vi "Idot Recorder.vi"() -> ()   [LabVIEW 2015]
uses:
  Libraries/NI-DAQ/NI-DAQ digitizer parameters.ctl
panel:
  in  "Parameters":T1={"physical channels"="Dev1/ai0:7", "input terminal configuration"=10106, "Range"=10.0, "Sample rate"=1000000.0, "samples per channel"=220000, "Trigger source"="/Dev1/PFI0", "pretrigger samples per channel"=20000, "task"="", "Sample mode"=10178, "Retriggerable"=FALSE} {"Sample mode" items=["Finite Samples"=10178, "Continuous Samples"=10123, "Hardware Timed Single Point"=12522]; "Sample rate" format="%.2p"; "input terminal configuration" items=["default"=-1, "RSE"=10083, "NRSE"=10078, "Differential"=10106, "Pseudodifferential"=12529]}
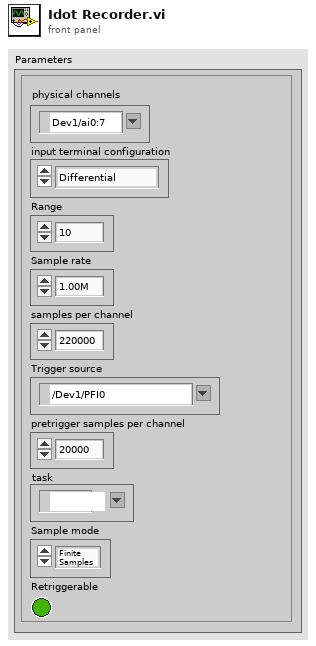
[diagram p1: front panel]
types:
  T1 = typedef "NI-DAQ digitizer parameters.ctl" = cluster{"physical channels":tag, "input terminal configuration":i32, "Range":dbl, "Sample rate":dbl, "samples per channel":i32, "Trigger source":tag, "pretrigger samples per channel":u32, "task":refnum<k21>, "Sample mode":i32, "Retriggerable":bool}
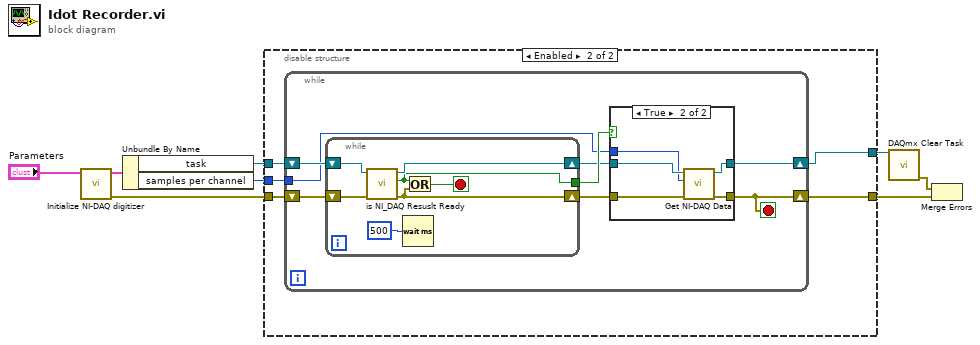
[diagram p0: block diagram]
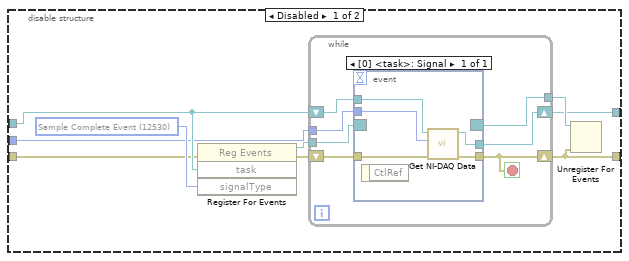
[diagram p2: hidden frame]
diagram:
  n1 = call "Initialize NI-DAQ digitizer.vi"("Parameters"="Parameters") -> ("error out"=w5:errorcluster, "Parameters out"=w7:T1)  [unwired: 9 in]
  n2 = Unbundle By Name(w7) -> ("task"=w6:refnum<k21>, "samples per channel"=w1:i32)
  n3 = disable-structure shown="Enabled" {
    disable-tunnel: w6 -> [w15 w34]
    disable-tunnel: w5 -> [w12 w33]
    disable-tunnel: [w11 w30] -> w3
    disable-tunnel: [w10 w31] -> w2
    disable-tunnel: w1 -> [w9 w32]
    frame Disabled {
      w16 = 12530 items=["Sample Complete Event"=12530, "Counter Output Event"=12494, "Change Detection Event"=12511, "Sample Clock"=12487] ("signalType")
      n4 = register-events(error in=w12, w15, w16) -> (reference out=w17:refnum<event-registration>, error out=w13:errorcluster)  [unwired: 1 in]
      n5 = while {
        tunnel: w17 -> [w24]
        shift-right: [w21] -> w10
        shift-left: w15 -> [w23]
        tunnel: [w22] -> w14
        shift-right: [w19] -> w11
        shift-left: w13 -> [w20]
        tunnel: w9 -> [w18]
        stop <- w19 stop-if-true
        n6 = event shown="[0] <task>: Signal" {
          selector: w24 -> [_]
          dyn-events: [_] -> w22
          timeout: _ -> [_]
          tunnel: w23 -> [w29]
          tunnel: [w28] -> w21
          tunnel: w20 -> [w27]
          tunnel: [w26] -> w19
          tunnel: w18 -> [w25]
          event Signal {
            n7 = event-data() -> ()  [unwired: 1 in, 1 out]
            n8 = call "Get NI-DAQ Data.vi"("error in (no error)"=w27, "samples per channel"=w25, "task"=w29) -> ("error out"=w26:errorcluster, "task out"=w28:refnum<k21>)  [unwired: 6 in, 1 out]
          }
        }
      }
      n9 = Unregister For Events(event registration refnum=w14, error in=w11) -> ()  [unwired: 1 out]
    }
    frame Enabled {
      n10 = while {
        shift-right: [w37] -> w31
        shift-left: w34 -> [w41]
        shift-right: [w36] -> w30
        shift-left: w33 -> [w42]
        tunnel: w32 -> [w35]
        stop <- w36 stop-if-true
        n11 = while {
          shift-right: [w53] -> w40
          shift-left: w42 -> [w56]
          shift-right: [w51] -> w38
          shift-left: w41 -> [w52]
          tunnel: [w50] -> w39
          stop <- w54 stop-if-true
          n12 = call "is NI_DAQ Resuslt Ready.vi"("error in (no error)"=w56, "task"=w52) -> ("error out"=w53:errorcluster, "Result Available"=w50:bool, "task out"=w51:refnum<k21>)  [unwired: 7 in]
          n13 = Wait (ms)(milliseconds to wait=u32 500) -> ()  [unwired: 1 out]
          n14 = Or(x=w50, y=w53) -> (x .or. y?=w54:bool)
        }
        n15 = case shown="True" w39 {
          tunnel: [w44 w49] -> w36
          tunnel: w40 -> [w44 w48]
          tunnel: w38 -> [w43 w47]
          tunnel: [w43 w46] -> w37
          tunnel: w35 -> [_ w45]
          frame False {
          }
          frame True {
            n16 = call "Get NI-DAQ Data.vi"("error in (no error)"=w48, "samples per channel"=w45, "task"=w47) -> ("error out"=w49:errorcluster, "task out"=w46:refnum<k21>)  [unwired: 6 in, 1 out]
          }
        }
      }
    }
  }
  n17 = call <vilib>:"DAQmx Clear Task.vi"("task in"=w2) -> ("error out"=w4:errorcluster)  [unwired: 14 in]
  n18 = Merge Errors(w4, w3) -> ()  [unwired: 1 out]
